vi "Get Test Interface Path.vi"(11 "Mock Class Generator Test in":refnum<class "Responsive Mock Class Generator Test.lvclass">) -> (3 "Test Class Path":path)   [LabVIEW 2020, in "Responsive Mock Class Generator Test.lvclass"]
uses:
  Responsive Mock Class Generator Test.lvclass
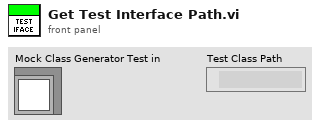
[diagram p1: front panel]
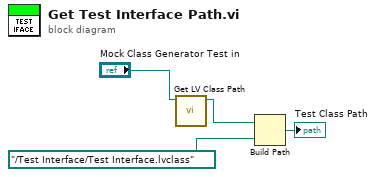
[diagram p0: block diagram]
diagram:
  n1 = call <vilib>:"Get LV Class Path.vi"("object"="Mock Class Generator Test in") -> ("class path"=w2:path)  [unwired: 9 in, 1 out]
  n2 = Build Path(base path=w2, name or relative path=path "../Test Interface/Test Interface.lvclass") -> (appended path=→"Test Class Path":path)
